vi "Command_Right_Joints.vi"(4 "Mode":enum32{"Position", "Velocity", "Effort"}(ring), 5 "node":string, 6 "error in":errorcluster, 9 "Goal":T1={"Label"="", "Arm Angles (degrees)"=[0.0, 0.0, 0.0, 0.0, 0.0, 0.0, 0.0]}) -> (0 "error out":errorcluster, 3 "JointCommand":T2={"Mode"=enum."Position", "Arm Angles"=[-0.7853981633974483, -0.7853981633974483, 0.0, 0.7853981633974483, 0.0, 1.5707963267948966, 0.0], "Angle Names"=["right_s0", "right_s1", "right_e0", "right_e1", "right_w0", "right_w1", "right_w2"]})   [LabVIEW 2013]
uses:
  ROS/RosMessages/Clusters/JointCommand.ctl
  Arm Globals.vi
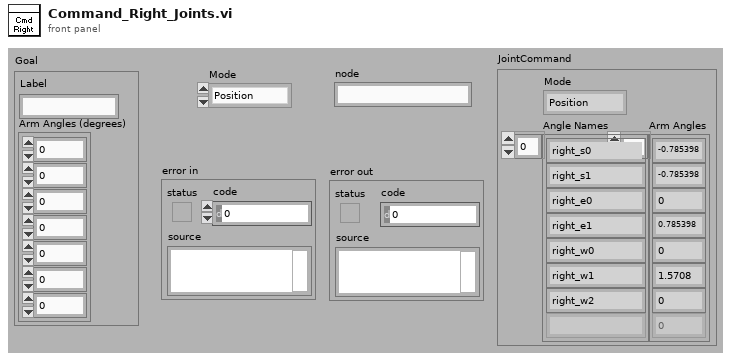
[diagram p1: front panel]
types:
  T1 = cluster{"Label":string, "Arm Angles (degrees)":dbl[]}
  T2 = typedef "JointCommand.ctl" = cluster{"Mode":enum32{"", "Position", "Velocity", "Effort"}, "Arm Angles":dbl[], "Angle Names":string[]}
  T3 = enum16{"big-endian, network order", "native, host order", "little-endian"}
  T4 = typedef "_ROSControl.ctl" = cluster{"topic port":u16, "Node":string, "topic":string, "type":string, "node port":u32, "error ":errorcluster, "Direction":T5, "APIs":string[]}
  T5 = typedef "_ROSDirection.ctl" = enum16{"Node", "Publisher", "Subscriber", "Service Client"}
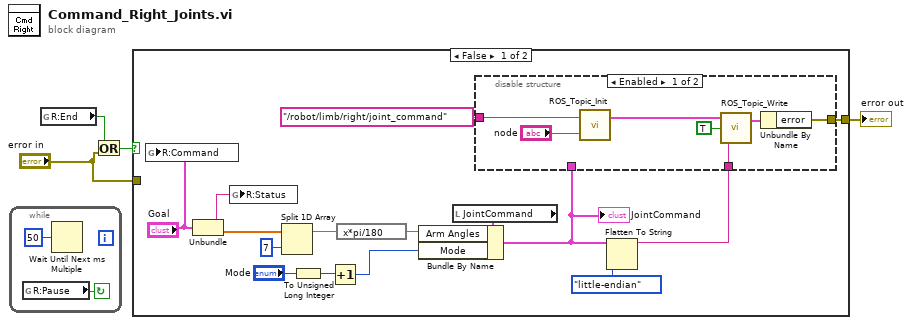
[diagram p0: block diagram]
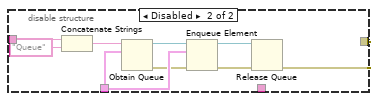
[diagram p2: hidden frame]
diagram:
  n1 = while {
    stop <- w6 continue-if-true
    n2 = global read "Arm Globals.vi" "R:Pause"() -> (w6:bool)
    n3 = Wait Until Next ms Multiple(millisecond multiple=u32 50) -> ()  [unwired: 1 out]
  }
  n4 = global read "Arm Globals.vi" "R:End"() -> (w3:bool)
  n5 = Or(x=w3, y="error in") -> (x .or. y?=w2:bool)
  n6 = case shown="False" w2 {
    tunnel: [w21 w38] -> w4
    tunnel: "error in" -> [_ w38]
    frame False {
      n7 = global write "Arm Globals.vi" "R:Command"("Goal") -> ()
      n8 = Unbundle("Goal") -> ("Label"=w8:string, "Arm Angles (degrees)"=w10:dbl[])
      n9 = global write "Arm Globals.vi" "R:Status"(w8) -> ()
      n10 = Split 1D Array(array=w10, index=7) -> (first subarray=w12:dbl[])  [unwired: 1 out]
      n11 = To Unsigned Long Integer(number="Mode") -> (unsigned 32bit integer=w14:u32)
      n12 = Increment(x=w14) -> (x+1=w16:u32)
      n13 = expression code="x*pi/180"(w12) -> (w15:dbl[])
      n14 = local read "JointCommand"() -> (w13:T2)
      n15 = Bundle By Name(cluster=w13, "Arm Angles"=w15, "Mode"=w16) -> (w7:T2)
      "JointCommand" <- w7
      n16 = Flatten To String(anything=w7, byte order (0:big-endian, network order)=T3."little-endian") -> (data string=w19:string)  [unwired: 2 in, 2 out]
      n17 = disable-structure shown="Enabled" {
        disable-tunnel: [w28 w29] -> w21
        disable-tunnel: w19 -> [w27 _]
        disable-tunnel: "/robot/limb/right/joint_command" ("topic") -> [w23 w37]
        disable-tunnel: w7 -> [_ w33]
        frame Enabled {
          n18 = call "ROS_Topic_Init.vi"("node"="node", "topic"=w23) -> ("ROS out"=w25:T4)  [unwired: 1 in]
          n19 = call "ROS_Topic_Write.vi"("Msg in"=w27, "Continuous?"=TRUE, "ROS in"=w25) -> ("ROS out"=w24:T4)  [unwired: 1 in]
          n20 = Unbundle By Name(w24) -> ("error"=w28:errorcluster)
        }
        frame Disabled {
          n21 = Concatenate Strings(w37, "Queue" ("string")) -> (w35:string)
          n22 = Obtain Queue(name (unnamed)=w35, element data type=w33) -> (queue out=w34:refnum<queue>, error out=w31:errorcluster)  [unwired: 3 in, 1 out]
          n23 = Enqueue Element(queue=w34, element=w33, error in (no error)=w31) -> (queue out=w32:refnum<queue>, error out=w30:errorcluster)  [unwired: 1 in, 1 out]
          n24 = Release Queue(queue=w32, error in (no error)=w30) -> (error out=w29:errorcluster)  [unwired: 1 in, 2 out]
        }
      }
    }
    frame True {
    }
  }
  "error out" <- w4
